vi "Set Intake Action.vi"(8 "error in":errorcluster, 11 "Action":T1=enum."Contain") -> (0 "error out":errorcluster)   [LabVIEW 2014]
uses:
  Intake Actions.ctl
  Intake Control.ctl
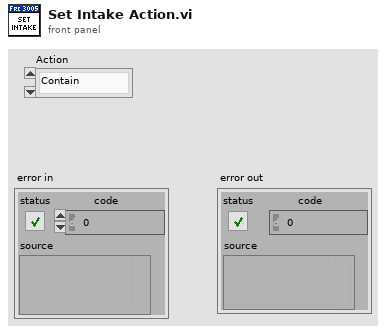
[diagram p1: front panel]
types:
  T1 = typedef "Intake Actions.ctl" = enum16{"Extend", "Contain", "Motor Still", "Motor Outward", "Motor Inward", "Collect", "Pass", "Herd", "Contain Off", "Collect Delay Off", "Patea"}
  T2 = typedef "Intake Control.ctl" = enum16{"Idle", "Contain", "Extend", "Motor Still", "Motor Outward", "Motor Inward", "Patea Extend", "Patea Retract"}
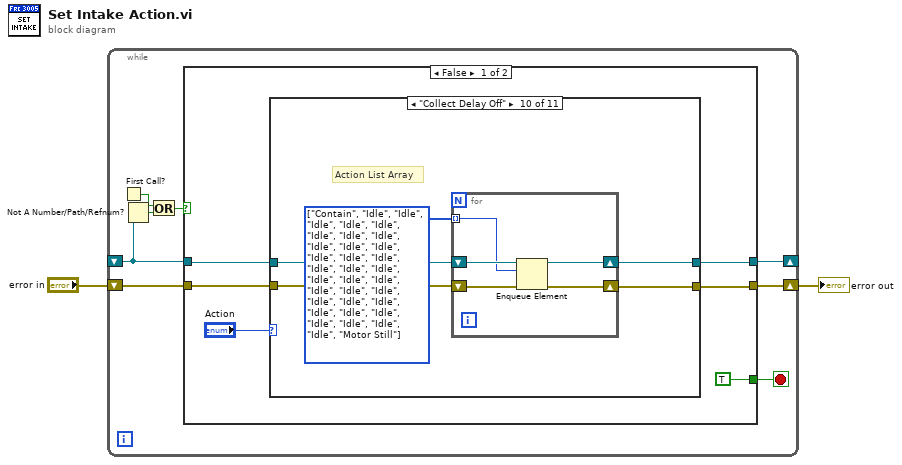
[diagram p0: block diagram]
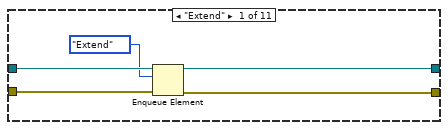
[diagram p2: hidden frame]
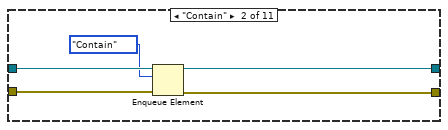
[diagram p3: hidden frame]
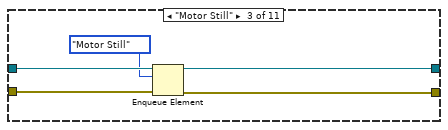
[diagram p4: hidden frame]
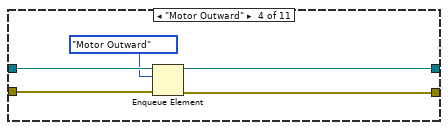
[diagram p5: hidden frame]
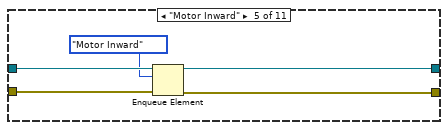
[diagram p6: hidden frame]
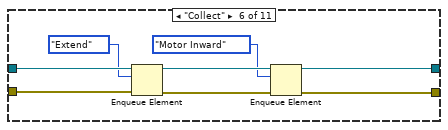
[diagram p7: hidden frame]
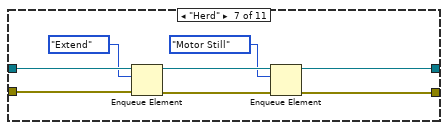
[diagram p8: hidden frame]
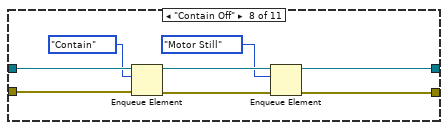
[diagram p9: hidden frame]
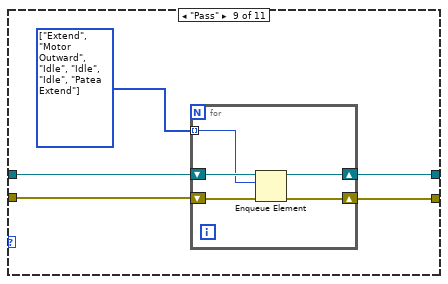
[diagram p10: hidden frame]
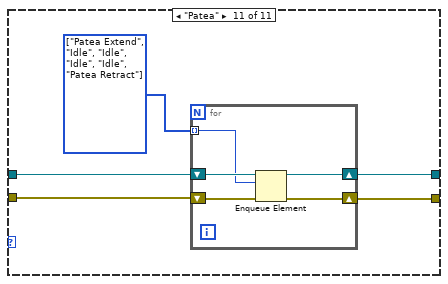
[diagram p11: hidden frame]
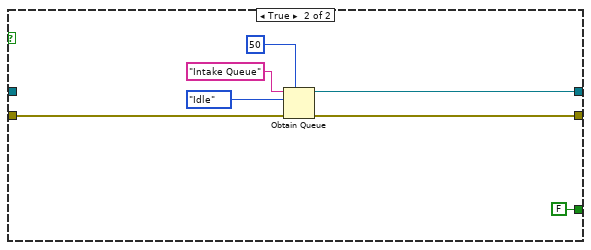
[diagram p12: hidden frame]
diagram:
  n1 = while {
    shift-right: [w10] -> _
    shift-left: _ -> [w6]
    shift-right: [w9] -> w2
    shift-left: "error in" -> [w7]
    stop <- w8 stop-if-true
    n2 = First Call?() -> (First Call?: T/F=w5:bool)
    n3 = Not A Number/Path/Refnum?(number/path/refnum=w6) -> (NaN/Path/Refnum?=w3:bool)
    n4 = Or(x=w5, y=w3) -> (x .or. y?=w4:bool)
    n5 = case shown="False" w4 {
      tunnel: [w13 w100] -> w10
      tunnel: [w14 w99] -> w9
      tunnel: [TRUE FALSE] -> w8
      tunnel: w6 -> [w16 _]
      tunnel: w7 -> [w12 w97]
      frame False {
        n6 = case shown="\"Collect Delay Off\"" "Action" {
          tunnel: w16 -> [w21 w26 w31 w36 w41 w49 w57 w65 w69 w79 w89]
          tunnel: [w19 w22 w29 w34 w39 w45 w53 w61 w67 w77 w87] -> w14
          tunnel: [w18 w23 w28 w33 w38 w43 w51 w59 w68 w78 w88] -> w13
          tunnel: w12 -> [w17 w24 w27 w32 w37 w46 w54 w62 w66 w76 w86]
          frame "Extend" {
            n7 = Enqueue Element(queue=w21, element=Intake_Control."Extend", error in (no error)=w17) -> (queue out=w18:refnum<queue>, error out=w19:errorcluster)  [unwired: 1 in, 1 out]
          }
          frame "Contain" {
            n8 = Enqueue Element(queue=w26, element=Intake_Control."Contain", error in (no error)=w24) -> (queue out=w23:refnum<queue>, error out=w22:errorcluster)  [unwired: 1 in, 1 out]
          }
          frame "Motor Still" {
            n9 = Enqueue Element(queue=w31, element=Intake_Control."Motor Still", error in (no error)=w27) -> (queue out=w28:refnum<queue>, error out=w29:errorcluster)  [unwired: 1 in, 1 out]
          }
          frame "Motor Outward" {
            n10 = Enqueue Element(queue=w36, element=Intake_Control."Motor Outward", error in (no error)=w32) -> (queue out=w33:refnum<queue>, error out=w34:errorcluster)  [unwired: 1 in, 1 out]
          }
          frame "Motor Inward" {
            n11 = Enqueue Element(queue=w41, element=Intake_Control."Motor Inward", error in (no error)=w37) -> (queue out=w38:refnum<queue>, error out=w39:errorcluster)  [unwired: 1 in, 1 out]
          }
          frame "Collect" {
            n12 = Enqueue Element(queue=w49, element=Intake_Control."Extend", error in (no error)=w46) -> (queue out=w44:refnum<queue>, error out=w47:errorcluster)  [unwired: 1 in, 1 out]
            n13 = Enqueue Element(queue=w44, element=Intake_Control."Motor Inward", error in (no error)=w47) -> (queue out=w43:refnum<queue>, error out=w45:errorcluster)  [unwired: 1 in, 1 out]
          }
          frame "Herd" {
            n14 = Enqueue Element(queue=w57, element=Intake_Control."Extend", error in (no error)=w54) -> (queue out=w52:refnum<queue>, error out=w55:errorcluster)  [unwired: 1 in, 1 out]
            n15 = Enqueue Element(queue=w52, element=Intake_Control."Motor Still", error in (no error)=w55) -> (queue out=w51:refnum<queue>, error out=w53:errorcluster)  [unwired: 1 in, 1 out]
          }
          frame "Contain Off" {
            n16 = Enqueue Element(queue=w65, element=Intake_Control."Contain", error in (no error)=w62) -> (queue out=w60:refnum<queue>, error out=w63:errorcluster)  [unwired: 1 in, 1 out]
            n17 = Enqueue Element(queue=w60, element=Intake_Control."Motor Still", error in (no error)=w63) -> (queue out=w59:refnum<queue>, error out=w61:errorcluster)  [unwired: 1 in, 1 out]
          }
          frame "Pass" {
            w70 = T2[] [enum."Extend", enum."Motor Outward", enum."Idle", enum."Idle", enum."Idle", enum."Patea Extend"] items=["Idle", "Contain", "Extend", "Motor Still", "Motor Outward", "Motor Inward", "Patea Extend", "Patea Retract"]
            n18 = for {
              tunnel: w70 -> [w71] mode=indexing
              shift-right: [w74] -> w68
              shift-left: w69 -> [w75]
              shift-right: [w73] -> w67
              shift-left: w66 -> [w72]
              n19 = Enqueue Element(queue=w75, element=w71, error in (no error)=w72) -> (queue out=w74:refnum<queue>, error out=w73:errorcluster)  [unwired: 1 in, 1 out]
            }
          }
          frame "Collect Delay Off" {
            w80 = T2[] [enum."Contain", enum."Idle", enum."Idle", enum."Idle", enum."Idle", enum."Idle", enum."Idle", enum."Idle", enum."Idle", enum."Idle", enum."Idle", enum."Idle", enum."Idle", enum."Idle", enum."Idle", enum."Idle", enum."Idle", enum."Idle", enum."Idle", enum."Idle", enum."Idle", enum."Idle", enum."Idle", enum."Idle", enum."Idle", enum."Idle", enum."Idle", enum."Idle", enum."Idle", enum."Idle", enum."Idle", enum."Idle", enum."Idle", enum."Idle", enum."Motor Still"] items=["Idle", "Contain", "Extend", "Motor Still", "Motor Outward", "Motor Inward", "Patea Extend", "Patea Retract"]
            # "Action List Array"
            n20 = for {
              tunnel: w80 -> [w81] mode=indexing
              shift-right: [w84] -> w78
              shift-left: w79 -> [w85]
              shift-right: [w83] -> w77
              shift-left: w76 -> [w82]
              n21 = Enqueue Element(queue=w85, element=w81, error in (no error)=w82) -> (queue out=w84:refnum<queue>, error out=w83:errorcluster)  [unwired: 1 in, 1 out]
            }
          }
          frame "Patea" {
            w90 = T2[] [enum."Patea Extend", enum."Idle", enum."Idle", enum."Idle", enum."Idle", enum."Patea Retract"] items=["Idle", "Contain", "Extend", "Motor Still", "Motor Outward", "Motor Inward", "Patea Extend", "Patea Retract"]
            n22 = for {
              tunnel: w90 -> [w91] mode=indexing
              shift-right: [w94] -> w88
              shift-left: w89 -> [w95]
              shift-right: [w93] -> w87
              shift-left: w86 -> [w92]
              n23 = Enqueue Element(queue=w95, element=w91, error in (no error)=w92) -> (queue out=w94:refnum<queue>, error out=w93:errorcluster)  [unwired: 1 in, 1 out]
            }
          }
        }
      }
      frame True {
        n24 = Obtain Queue(max queue size (-1, unlimited)=50, name (unnamed)="Intake Queue", element data type=Intake_Control."Idle", error in (no error)=w97) -> (queue out=w100:refnum<queue>, error out=w99:errorcluster)  [unwired: 1 in, 1 out]
      }
    }
  }
  "error out" <- w2
